vi "Helmholtz2D_FEM_Solver.vi"(0 "F(x, y)":dbl[](array[numeric]), 1 "Grid":cluster{"Xi":dbl[], "Yi":dbl[]}, 5 "k":dbl=1.0, 7 "a":dbl, 9 "Domain":cluster{"X":dbl[], "Y":dbl[]}, 11 "error in (no error)":errorcluster, 12 "Boundary Condition":cluster{"type":T1, "Value":dbl[]} {"type" items=["Dirichlet", "Neumann"]}) -> (4 "U(x, y)":dbl[](array[numeric]), 6 "X Used":dbl[](array[numeric]), 8 "Y Used":dbl[](array[numeric]), 10 "Triangulation":i32[][](array[numeric]), 15 "error out":errorcluster)   [LabVIEW 2017, in "NI_PDE.lvlib"]
uses:
  <vilib>/gmath/NI_PDE.lvlib
  <vilib>/gmath/pde.llb/Common/PDE_BC Type.ctl
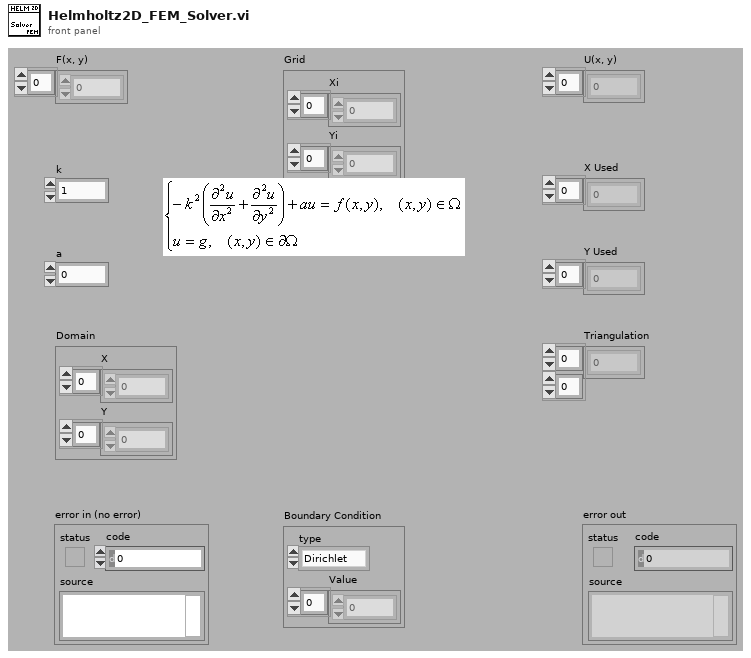
[diagram p1: front panel]
types:
  T1 = typedef "NI_PDE.lvlib/PDE_BC Type.ctl" = i32
  T2 = typedef "NI_PDE.lvlib/Helmholtz2D_FEM_Data.ctl" = cluster{"PDE":cluster{"k":dbl, "a":dbl, "F(x, y)":dbl[]}, "# of unknown":i32, "# of known":i32, "U(x, y)":dbl[], "X Used":dbl[], "Y Used":dbl[], "Triangulation":i32[][], "Coef Mtrx":T3}
  T3 = typedef "NI_PDE.lvlib/PDE_Sparse Mtrx.ctl" = cluster{"Row":cluster{"col":i32, "value":dbl}[]}[]
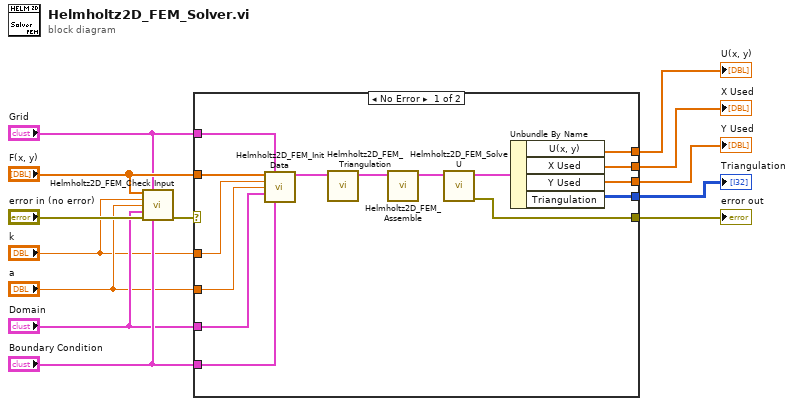
[diagram p0: block diagram]
diagram:
  n1 = call <vilib>:"Helmholtz2D_FEM_Check Input.vi"("F(x, y)"="F(x, y)", "Grid"="Grid", "k"="k", "a"="a", "Domain"="Domain", "error in (no error)"="error in (no error)", "Boundary Condition"="Boundary Condition") -> ("error out"=w12:errorcluster)  [unwired: 8 out]
  n2 = case shown="No Error" w12 {
    selector: w12 -> [_ w29]
    tunnel: [w15 w29] -> w11
    tunnel: "Boundary Condition" -> [w25 _]
    tunnel: "Domain" -> [w26 _]
    tunnel: "a" -> [w16 _]
    tunnel: "k" -> [w27 _]
    tunnel: "F(x, y)" -> [w28 _]
    tunnel: "Grid" -> [w24 _]
    tunnel: [w19 _] -> w2
    tunnel: [w18 _] -> w3
    tunnel: [w17 _] -> w4
    tunnel: [w14 _] -> w1
    frame No Error {
      n3 = call <vilib>:"Helmholtz2D_FEM_Init Data.vi"("F(x, y)"=w28, "Grid"=w24, "k"=w27, "a"=w16, "Domain"=w26, "Boundary Condition"=w25) -> ("Helmholtz2D FEM Data"=w23:T2)  [unwired: 9 out]
      n4 = call <vilib>:"Helmholtz2D_FEM_Triangulation.vi"("Helmholtz2D FEM Data In"=w23) -> ("Helmholtz2D FEM Data Out"=w22:T2)  [unwired: 10 out]
      n5 = call <vilib>:"Helmholtz2D_FEM_Assemble.vi"("Helmholtz2D FEM Data In"=w22) -> ("Helmholtz2D FEM Data Out"=w21:T2)  [unwired: 10 out]
      n6 = call <vilib>:"Helmholtz2D_FEM_Solve U.vi"("Helmholtz2D FEM Data In"=w21) -> ("error out"=w15:errorcluster, "Helmholtz2D FEM Data Out"=w20:T2)  [unwired: 1 in, 8 out]
      n7 = Unbundle By Name(w20) -> ("U(x, y)"=w14:dbl[], "X Used"=w19:dbl[], "Y Used"=w18:dbl[], "Triangulation"=w17:i32[][])
    }
    frame Error {
    }
  }
  "U(x, y)" <- w1
  "error out" <- w11
  "X Used" <- w2
  "Y Used" <- w3
  "Triangulation" <- w4
